vi "Inverse Dynamics (Point).vi"(0 "serial arm in":refnum<class "NI_Robotics_Serial Robot Arm.lvclass">, 1 "external force":dbl[](array[numeric])=[0.0, 0.0, 0.0, 0.0, 0.0, 0.0], 2 "gravity":dbl[](array[numeric]), 5 "joint positions":dbl[](array[numeric]), 7 "joint velocities":dbl[](array[numeric]), 9 "joint accelerations":dbl[](array[numeric]), 11 "error in (no error)":errorcluster) -> (4 "serial arm out":refnum<class "NI_Robotics_Serial Robot Arm.lvclass">, 6 "required torques":dbl[](array[numeric]), 15 "error out":errorcluster)   [LabVIEW 2017, in "NI_Kinematics.lvlib"]
doc: "Returns the amount of torque required for the robotic arm to achieve the joint positions, velocities, and accelerations you specify. Wire data to the <B>joint positions</B> input to determine the polymorphic instance to use or manually select the instance.\n\n<B>.m file:</B> rne"
uses:
  <vilib>/robotics/Kinematics/NI_Kinematics.lvlib
  <vilib>/robotics/Kinematics/Robot/NI_Robotics_Serial Robot Arm.lvclass
  <vilib>/Analysis/Matrix/Datatypes/RealMatrix.ctl
  <vilib>/robotics/Kinematics/Link/Joint Type.ctl
  <vilib>/Analysis/baseanly.llb/Real A x B.vi
  <vilib>/Analysis/baseanly.llb/A x Vector.vi
  <vilib>/Analysis/baseanly.llb/Real Dot Product.vi
  <vilib>/Analysis/Matrix/Numeric/Conversions/Array To Matrix - RA2.vi
  <vilib>/robotics/Kinematics/Link/NI_Robotics_Link.lvclass
  <vilib>/Analysis/NI_AALBase.lvlib
  <vilib>/Analysis/NI_AALPro.lvlib
  <vilib>/Analysis/Matrix/NI_Matrix.lvlib
  <vilib>/robotics/Utilities/NI_Robotics Utilities.lvlib
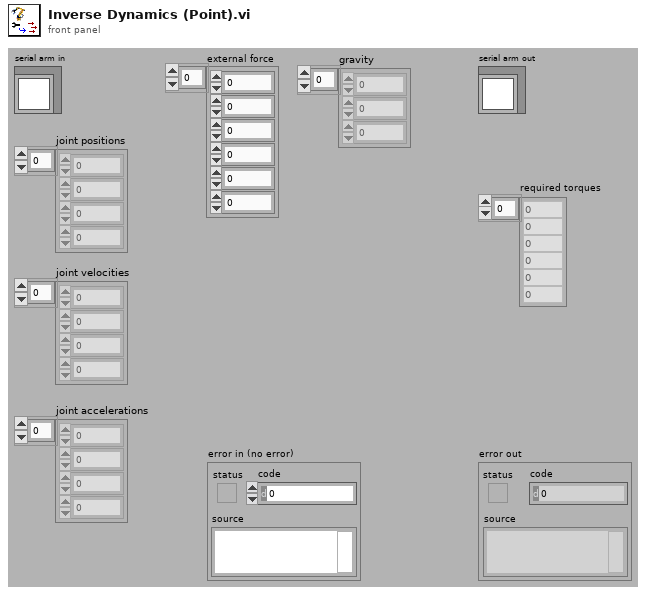
[diagram p1: front panel]
types:
  T1 = typedef "NI_Matrix.lvlib/RealMatrix.ctl" = dbl[][]
  T2 = typedef "NI_Robotics_Link.lvclass/Joint Type.ctl" = enum16{"Revolute", "Prismatic"}
  T3 = typedef "NI_Kinematics.lvlib/DH Convention.ctl" = enum16{"Standard", "Modified"}
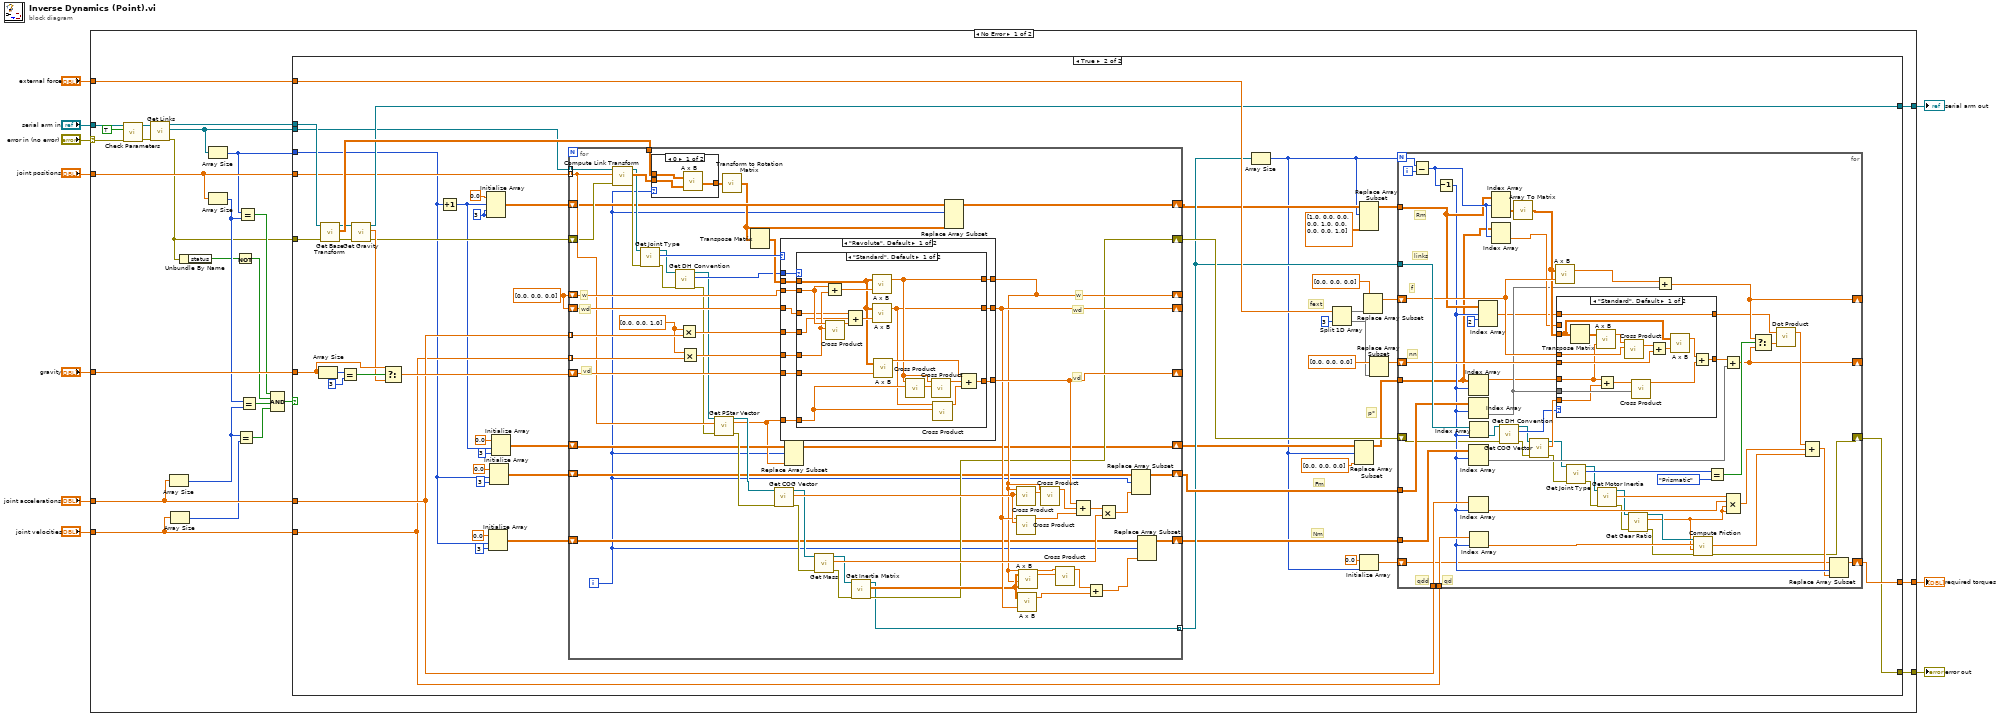
[diagram p0: block diagram]
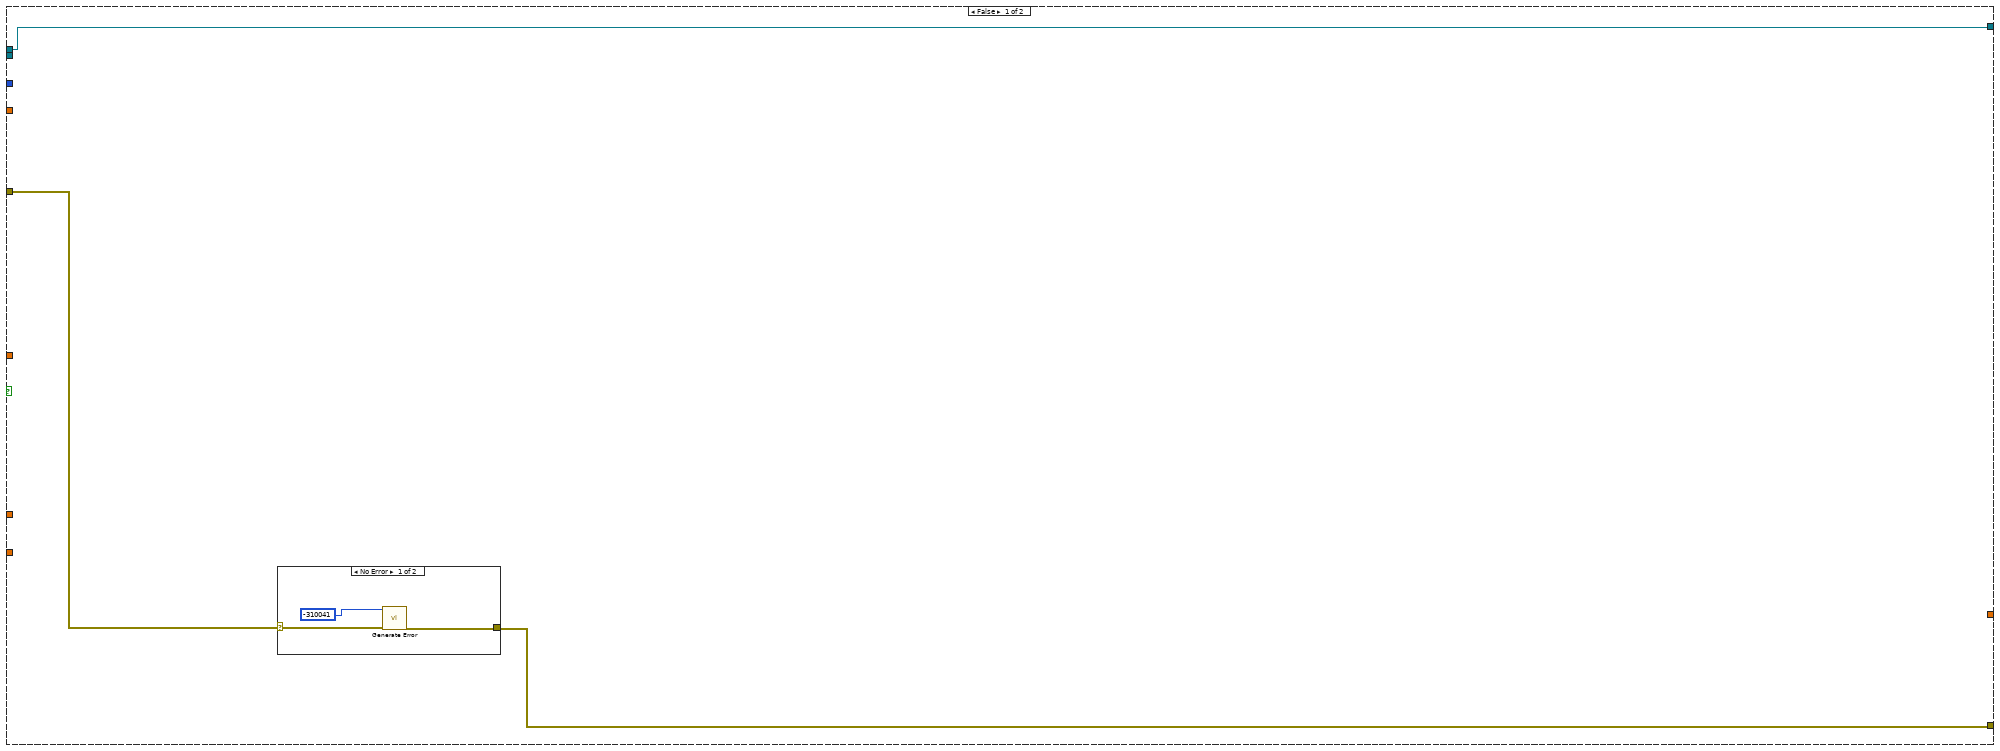
[diagram p2: hidden frame]
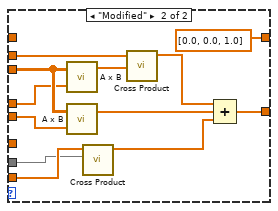
[diagram p4: hidden frame]
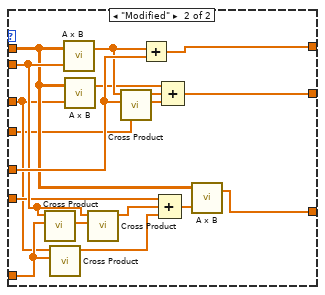
[diagram p5: hidden frame]
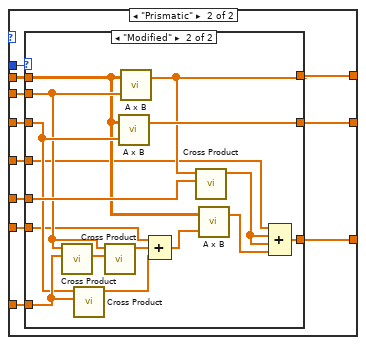
[diagram p6: hidden frame]
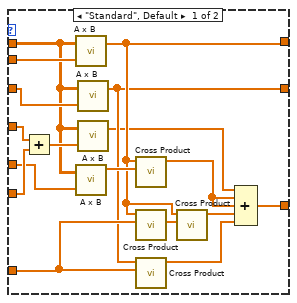
[diagram p7: hidden frame]
diagram:
  n1 = case shown="No Error" "error in (no error)" {
    selector: "error in (no error)" -> [w12 w331]
    tunnel: "external force" -> [w36 _]
    tunnel: [w35 _] -> w9
    tunnel: "gravity" -> [w34 _]
    tunnel: [w32 w332] -> w7
    tunnel: "joint positions" -> [w31 _]
    tunnel: "joint accelerations" -> [w30 _]
    tunnel: "joint velocities" -> [w29 _]
    tunnel: [w23 w331] -> w3
    tunnel: "serial arm in" -> [w17 w332]
    frame No Error {
      n2 = call <vilib>:"Check Parameters.vi"("error in (no error)"=w12, "Dynamic Model"=TRUE, "NI_Robotics_Serial Robot Arm in"=w17) -> ("error out"=w15:errorcluster, "NI_Robotics_Serial Robot Arm out"=w16:refnum<class "NI_Robotics_Serial Robot Arm.lvclass">)  [unwired: 7 in]
      n3 = call <vilib>:"Get Links.vi"("error in (no error)"=w15, "serial arm in"=w16) -> ("error out"=w14:errorcluster, "links"=w28:refnum<class "NI_Robotics_Link.lvclass">[], "serial arm out"=w33:refnum<class "NI_Robotics_Serial Robot Arm.lvclass">)  [unwired: 7 in]
      n4 = Array Size(array=w30) -> (size(s)=w25:i32)
      n5 = Array Size(array=w29) -> (size(s)=w27:i32)
      n6 = Unbundle By Name(w14) -> ("status"=w20:bool)
      n7 = Array Size(array=w31) -> (size(s)=w26:i32)
      n8 = Array Size(array=w28) -> (size(s)=w11:i32)
      n9 = Not(x=w20) -> (.not. x?=w19:bool)
      n10 = Equal?(x=w25, y=w27) -> (x = y?=w22:bool)
      n11 = Equal?(x=w11, y=w26) -> (x = y?=w18:bool)
      n12 = Equal?(x=w26, y=w25) -> (x = y?=w21:bool)
      n13 = Compound Arithmetic op=AND(w18, w19, w21, w22) -> (w24:bool)
      n14 = case shown="True" w24 {
        tunnel: w36 -> [_ w97]
        tunnel: [_ w93] -> w35
        tunnel: w34 -> [_ w89]
        tunnel: w33 -> [w39 w85]
        tunnel: [w39 w83] -> w32
        tunnel: w31 -> [_ w82]
        tunnel: w30 -> [_ w81]
        tunnel: w29 -> [_ w80]
        tunnel: w28 -> [_ w79]
        tunnel: [w37 w74] -> w23
        tunnel: w14 -> [w38 w78]
        tunnel: w11 -> [_ w64]
        frame False {
          n15 = case shown="No Error" w38 {
            selector: w38 -> [w42 w43]
            tunnel: [w41 w43] -> w37
            frame No Error {
              n16 = call <vilib>:"Generate Error.vi"("error in (no error)"=w42, "code"=-310041) -> ("error out"=w41:errorcluster)  [unwired: 9 in]
            }
            frame Error {
              # "propagate error"
            }
          }
        }
        frame True {
          w72 = 3 ("dimension size")
          w98 = dbl[] [0.0, 0.0, 0.0]
          # "fext"
          # "p*"
          # "Nm"
          # "Fm"
          n17 = Array Size(array=w89) -> (size(s)=w91:i32)
          n18 = call <vilib>:"Get Base Transform.vi"("error in (no error)"=w78, "serial arm in"=w85) -> ("error out"=w77:errorcluster, "base transform"=w87:T1, "serial arm out"=w84:refnum<class "NI_Robotics_Serial Robot Arm.lvclass">)  [unwired: 7 in]
          n19 = Equal?(x=w91, y=3) -> (x = y?=w92:bool)
          n20 = call <vilib>:"Get Gravity.vi"("error in (no error)"=w77, "serial arm in"=w84) -> ("error out"=w76:errorcluster, "gravity"=w86:dbl[], "serial arm out"=w83:refnum<class "NI_Robotics_Serial Robot Arm.lvclass">)  [unwired: 7 in]
          n21 = Select(t=w89, s=w92, f=w86) -> (s? t:f=w88:dbl[])
          n22 = Increment(x=w64) -> (x+1=w71:i32)
          n23 = Initialize Array(0.0 ("element"), w71, w72, w72) -> (w63:dbl[][][])
          n24 = Initialize Array(0.0 ("element"), w64, 3 ("dimension size")) -> (w59:dbl[][])
          n25 = Initialize Array(0.0 ("element"), w64, 3 ("dimension size")) -> (w61:dbl[][])
          n26 = Initialize Array(0.0 ("element"), w71, 3 ("dimension size")) -> (w62:dbl[][])
          n27 = for {
            tunnel: w82 -> [w211] mode=indexing
            tunnel: w79 -> [w208] mode=indexing
            tunnel: w87 -> [w236]
            shift-right: [w215] -> _
            shift-left: w98 -> [w225]
            shift-right: [w217] -> _
            shift-left: w98 -> [w224]
            shift-right: [w222] -> _
            shift-left: w88 -> [w232]
            tunnel: w80 -> [w230] mode=indexing
            tunnel: w81 -> [w228] mode=indexing
            shift-right: [w195] -> w75
            shift-left: w76 -> [w209]
            shift-right: [w193] -> w50
            shift-left: w63 -> [w194]
            shift-right: [w189] -> w47
            shift-left: w62 -> [w191]
            shift-right: [w186] -> w60
            shift-left: w61 -> [w187]
            shift-right: [w184] -> w57
            shift-left: w59 -> [w185]
            tunnel: [w182] -> w58 mode=indexing
            i -> [w181]
            w227 = dbl[] [0.0, 0.0, 1.0]
            # "vd"
            # "wd"
            # "w"
            # "vd"
            # "wd"
            # "w"
            n28 = call <vilib>:"Compute Link Transform.vi"("error in (no error)"=w209, "q"=w211, "Link in"=w208) -> ("error out"=w205:errorcluster, "Link Transform"=w237:T1, "Link out"=w207:refnum<class "NI_Robotics_Link.lvclass">)  [unwired: 6 out]
            n29 = call <vilib>:"Get Joint Type.vi"("error in (no error)"=w205, "Link in"=w207) -> ("error out"=w203:errorcluster, "Joint Type"=w234:T2, "Link out"=w206:refnum<class "NI_Robotics_Link.lvclass">)  [unwired: 7 in]
            n30 = case shown="0" w181 {
              tunnel: w237 -> [w328 w330]
              tunnel: [w327 w330] -> w235
              tunnel: w236 -> [w329 _]
              frame 0 {
                n31 = call-poly <vilib>:"A x B.vi"("B"=w328, "A"=w329) -> ("A x B"=w327:T1)  [unwired: 1 out]
              }
              frame 1, Default {
              }
            }
            n32 = call <vilib>:"Get DH Convention.vi"("error in (no error)"=w203, "Link In"=w206) -> ("error out"=w202:errorcluster, "DH Convention"=w210:T3, "Link Out"=w204:refnum<class "NI_Robotics_Link.lvclass">)  [unwired: 7 in]
            n33 = Multiply(x=w227, y=w228) -> (x*y=w229:dbl[])
            n34 = Multiply(x=w227, y=w230) -> (x*y=w231:dbl[])
            n35 = call <vilib>:"Get PStar Vector.vi"("error in (no error)"=w202, "q"=w211, "link in"=w204) -> ("error out"=w198:errorcluster, "p*"=w190:dbl[], "link out"=w201:refnum<class "NI_Robotics_Link.lvclass">)  [unwired: 6 in]
            n36 = call <vilib>:"Transform to Rotation Matrix.vi"("transform"=w235) -> ("rotation matrix"=w192:T1)
            n37 = Transpose Matrix(1:w192) -> (0:w233:T1)
            n38 = call <vilib>:"Get COG Vector.vi"("error in (no error)"=w198, "Link.lvclass in"=w201) -> ("error out"=w197:errorcluster, "COG Vector"=w223:dbl[], "Link.lvclass out"=w200:refnum<class "NI_Robotics_Link.lvclass">)  [unwired: 7 in]
            n39 = case shown="\"Revolute\", Default" w234 {
              tunnel: w233 -> [w246 w288]
              tunnel: w225 -> [w248 w289]
              tunnel: w224 -> [w243 w290]
              tunnel: [w240 w285] -> w215
              tunnel: [w239 w284] -> w217
              tunnel: w229 -> [w242 w291]
              tunnel: w231 -> [w244 w287]
              tunnel: w232 -> [w245 w292]
              tunnel: w190 -> [w241 w286]
              tunnel: [w247 w293] -> w222
              tunnel: w210 -> [w238 w283]
              frame "Revolute", Default {
                n40 = case shown="\"Standard\", Default" w238 {
                  tunnel: w248 -> [w262 w275]
                  tunnel: [w261 w274] -> w247
                  tunnel: w246 -> [w258 w273]
                  tunnel: w245 -> [w257 w271]
                  tunnel: w244 -> [w256 w279]
                  tunnel: w243 -> [w255 w269]
                  tunnel: w242 -> [w254 w266]
                  tunnel: w241 -> [w252 w281]
                  tunnel: [w250 w280] -> w240
                  tunnel: [w249 w278] -> w239
                  frame "Standard", Default {
                    n41 = Add(x=w262, y=w256) -> (x+y=w263:dbl[])
                    n42 = call <vilib>:"Cross Product.vi"("B Vector"=w256, "A Vector"=w262) -> ("Cross Product"=w264:dbl[])  [unwired: 8 in, 1 out]
                    n43 = Compound Arithmetic op=ADD(w255, w254, w264) -> (w265:dbl[])
                    n44 = call-poly <vilib>:"A x B.vi"("Vector"=w263, "A"=w258) -> ("A x Vector"=w250:dbl[])  [unwired: 1 out]
                    n45 = call-poly <vilib>:"A x B.vi"("Vector"=w265, "A"=w258) -> ("A x Vector"=w249:dbl[])  [unwired: 1 out]
                    n46 = call-poly <vilib>:"A x B.vi"("Vector"=w257, "A"=w258) -> ("A x Vector"=w259:dbl[])  [unwired: 1 out]
                    n47 = call <vilib>:"Cross Product.vi"("B Vector"=w252, "A Vector"=w250) -> ("Cross Product"=w253:dbl[])  [unwired: 8 in, 1 out]
                    n48 = call <vilib>:"Cross Product.vi"("B Vector"=w253, "A Vector"=w250) -> ("Cross Product"=w251:dbl[])  [unwired: 8 in, 1 out]
                    n49 = call <vilib>:"Cross Product.vi"("B Vector"=w252, "A Vector"=w249) -> ("Cross Product"=w260:dbl[])  [unwired: 8 in, 1 out]
                    n50 = Compound Arithmetic op=ADD(w259, w251, w260) -> (w261:dbl[])
                  }
                  frame "Modified" {
                    n51 = call <vilib>:"Cross Product.vi"("B Vector"=w281, "A Vector"=w275) -> ("Cross Product"=w282:dbl[])  [unwired: 8 in, 1 out]
                    n52 = call <vilib>:"Cross Product.vi"("B Vector"=w281, "A Vector"=w269) -> ("Cross Product"=w268:dbl[])  [unwired: 8 in, 1 out]
                    n53 = call-poly <vilib>:"A x B.vi"("Vector"=w275, "A"=w273) -> ("A x Vector"=w277:dbl[])  [unwired: 1 out]
                    n54 = call-poly <vilib>:"A x B.vi"("Vector"=w269, "A"=w273) -> ("A x Vector"=w276:dbl[])  [unwired: 1 out]
                    n55 = call <vilib>:"Cross Product.vi"("B Vector"=w282, "A Vector"=w275) -> ("Cross Product"=w270:dbl[])  [unwired: 8 in, 1 out]
                    n56 = call <vilib>:"Cross Product.vi"("B Vector"=w279, "A Vector"=w277) -> ("Cross Product"=w267:dbl[])  [unwired: 8 in, 1 out]
                    n57 = Add(x=w277, y=w279) -> (x+y=w280:dbl[])
                    n58 = Compound Arithmetic op=ADD(w271, w270, w268) -> (w272:dbl[])
                    n59 = Compound Arithmetic op=ADD(w276, w267, w266) -> (w278:dbl[])
                    n60 = call-poly <vilib>:"A x B.vi"("Vector"=w272, "A"=w273) -> ("A x Vector"=w274:dbl[])  [unwired: 1 out]
                  }
                }
              }
              frame "Prismatic" {
                n61 = case shown="\"Modified\"" w283 {
                  tunnel: [w310 w326] -> w293
                  tunnel: w292 -> [w309 w313]
                  tunnel: w291 -> [w308 w314]
                  tunnel: w290 -> [w306 w321]
                  tunnel: w289 -> [w305 w320]
                  tunnel: w288 -> [w303 w319]
                  tunnel: w287 -> [w302 w322]
                  tunnel: w286 -> [w300 w324]
                  tunnel: [w299 w317] -> w285
                  tunnel: [w298 w323] -> w284
                  frame "Standard", Default {
                    n62 = Add(x=w308, y=w309) -> (x+y=w307:dbl[])
                    n63 = call-poly <vilib>:"A x B.vi"("Vector"=w305, "A"=w303) -> ("A x Vector"=w299:dbl[])  [unwired: 1 out]
                    n64 = call-poly <vilib>:"A x B.vi"("Vector"=w302, "A"=w303) -> ("A x Vector"=w304:dbl[])  [unwired: 1 out]
                    n65 = call-poly <vilib>:"A x B.vi"("Vector"=w306, "A"=w303) -> ("A x Vector"=w298:dbl[])  [unwired: 1 out]
                    n66 = call-poly <vilib>:"A x B.vi"("Vector"=w307, "A"=w303) -> ("A x Vector"=w294:dbl[])  [unwired: 1 out]
                    n67 = call <vilib>:"Cross Product.vi"("B Vector"=w304, "A Vector"=w299) -> ("Cross Product"=w295:dbl[])  [unwired: 8 in, 1 out]
                    n68 = call <vilib>:"Cross Product.vi"("B Vector"=w300, "A Vector"=w299) -> ("Cross Product"=w301:dbl[])  [unwired: 8 in, 1 out]
                    n69 = call <vilib>:"Cross Product.vi"("B Vector"=w300, "A Vector"=w298) -> ("Cross Product"=w297:dbl[])  [unwired: 8 in, 1 out]
                    n70 = call <vilib>:"Cross Product.vi"("B Vector"=w301, "A Vector"=w299) -> ("Cross Product"=w296:dbl[])  [unwired: 8 in, 1 out]
                    n71 = Compound Arithmetic op=ADD(w294, w295, w295, w296, w297) -> (w310:dbl[])
                  }
                  frame "Modified" {
                    n72 = call <vilib>:"Cross Product.vi"("B Vector"=w324, "A Vector"=w320) -> ("Cross Product"=w325:dbl[])  [unwired: 8 in, 1 out]
                    n73 = call <vilib>:"Cross Product.vi"("B Vector"=w324, "A Vector"=w321) -> ("Cross Product"=w315:dbl[])  [unwired: 8 in, 1 out]
                    n74 = call <vilib>:"Cross Product.vi"("B Vector"=w325, "A Vector"=w320) -> ("Cross Product"=w316:dbl[])  [unwired: 8 in, 1 out]
                    n75 = call-poly <vilib>:"A x B.vi"("Vector"=w321, "A"=w319) -> ("A x Vector"=w323:dbl[])  [unwired: 1 out]
                    n76 = call-poly <vilib>:"A x B.vi"("Vector"=w320, "A"=w319) -> ("A x Vector"=w317:dbl[])  [unwired: 1 out]
                    n77 = Compound Arithmetic op=ADD(w313, w316, w315) -> (w318:dbl[])
                    n78 = call <vilib>:"Cross Product.vi"("B Vector"=w322, "A Vector"=w317) -> ("Cross Product"=w311:dbl[])  [unwired: 8 in, 1 out]
                    n79 = call-poly <vilib>:"A x B.vi"("Vector"=w318, "A"=w319) -> ("A x Vector"=w312:dbl[])  [unwired: 1 out]
                    n80 = Compound Arithmetic op=ADD(w314, w311, w311, w312) -> (w326:dbl[])
                  }
                }
              }
            }
            n81 = Replace Array Subset(array=w191, new element=w190, index (row)=w181) -> (w189:dbl[][])  [unwired: 1 in]
            n82 = call <vilib>:"Get Mass.vi"("error in (no error)"=w197, "Link in"=w200) -> ("error out"=w196:errorcluster, "Mass"=w219:dbl, "Link out"=w199:refnum<class "NI_Robotics_Link.lvclass">)  [unwired: 7 in]
            n83 = call <vilib>:"Get Inertia Matrix.vi"("error in (no error)"=w196, "Link"=w199) -> ("error out"=w195:errorcluster, "Inertia Matrix"=w216:T1, "Link 2"=w182:refnum<class "NI_Robotics_Link.lvclass">)  [unwired: 7 in]
            n84 = Replace Array Subset(array=w194, new element=w192, index (dim 0)=w181) -> (w193:dbl[][][])  [unwired: 2 in]
            n85 = call <vilib>:"Cross Product.vi"("B Vector"=w223, "A Vector"=w215) -> ("Cross Product"=w226:dbl[])  [unwired: 8 in, 1 out]
            n86 = call <vilib>:"Cross Product.vi"("B Vector"=w223, "A Vector"=w217) -> ("Cross Product"=w220:dbl[])  [unwired: 8 in, 1 out]
            n87 = call-poly <vilib>:"A x B.vi"("Vector"=w217, "A"=w216) -> ("A x Vector"=w213:dbl[])  [unwired: 1 out]
            n88 = call-poly <vilib>:"A x B.vi"("Vector"=w215, "A"=w216) -> ("A x Vector"=w214:dbl[])  [unwired: 1 out]
            n89 = call <vilib>:"Cross Product.vi"("B Vector"=w226, "A Vector"=w215) -> ("Cross Product"=w221:dbl[])  [unwired: 8 in, 1 out]
            n90 = call <vilib>:"Cross Product.vi"("B Vector"=w214, "A Vector"=w215) -> ("Cross Product"=w212:dbl[])  [unwired: 8 in, 1 out]
            n91 = Compound Arithmetic op=ADD(w222, w221, w220) -> (w218:dbl[])
            n92 = Add(x=w212, y=w213) -> (x+y=w183:dbl[])
            n93 = Multiply(x=w218, y=w219) -> (x*y=w188:dbl[])
            n94 = Replace Array Subset(array=w187, new element=w188, index (row)=w181) -> (w186:dbl[][])  [unwired: 1 in]
            n95 = Replace Array Subset(array=w185, new element=w183, index (row)=w181) -> (w184:dbl[][])  [unwired: 1 in]
          }
          n96 = Array Size(array=w58) -> (size(s)=w44:i32)
          n97 = Split 1D Array(array=w97, index=3) -> (first subarray=w55:dbl[], second subarray=w51:dbl[])
          n98 = Replace Array Subset(array=w47, new element=dbl[] [0.0, 0.0, 0.0], index (row)=w44) -> (w46:dbl[][])  [unwired: 1 in]
          n99 = Replace Array Subset(array=w50, new element=T1 [[1.0, 0.0, 0.0], [0.0, 1.0, 0.0], [0.0, 0.0, 1.0]] ("Real Matrix"), index (dim 0)=w44) -> (w49:dbl[][][])  [unwired: 2 in]
          n100 = Initialize Array(0.0 ("element"), w44) -> (w94:dbl[])
          n101 = Replace Array Subset(array=dbl[] [0.0, 0.0, 0.0], new element=w55) -> (w54:dbl[])  [unwired: 1 in]
          n102 = Replace Array Subset(array=dbl[] [0.0, 0.0, 0.0], new element=w51) -> (w53:dbl[])  [unwired: 1 in]
          n103 = for {
            N: w44 -> [w153]
            tunnel: w49 -> [w143]
            tunnel: w58 -> [w151]
            tunnel: w46 -> [w115]
            shift-right: [w130] -> _
            shift-left: w53 -> [w145]
            shift-right: [w141] -> _
            shift-left: w54 -> [w146]
            tunnel: w60 -> [w149]
            tunnel: w57 -> [w148]
            shift-right: [w142] -> w93
            shift-left: w94 -> [w114]
            tunnel: w81 -> [w139]
            tunnel: w80 -> [w138]
            shift-right: [w102] -> w74
            shift-left: w75 -> [w111]
            i -> [w152]
            # "qd"
            # "qdd"
            # "f"
            # "nn"
            # "Rm"
            # "links"
            n104 = Subtract(x=w153, y=w152) -> (x-y=w150:i32)
            n105 = Decrement(x=w150) -> (x-1=w137:i32)
            n106 = Index Array(array=w115, index (row)=w137) -> (element=w116:dbl[])  [unwired: 1 in]
            n107 = Index Array(array=w149, index (row)=w137) -> (element=w124:dbl[])  [unwired: 1 in]
            n108 = Index Array(array=w148, index (row)=w137) -> (element=w131:dbl[])  [unwired: 1 in]
            n109 = Index Array(array=w139, index=w137) -> (element=w118:dbl)
            n110 = Index Array(array=w151, index=w137) -> (element=w126:refnum<class "NI_Robotics_Link.lvclass">)
            n111 = Index Array(array=w138, index=w137) -> (element=w136:dbl)
            n112 = Index Array(array=w143, index (dim 0)=w137, index (dim 1)=2 ("index (row)")) -> (element=w120:dbl[])  [unwired: 1 in]
            n113 = Index Array(array=w143, index (dim 0)=w150) -> (element=w101:dbl[][])  [unwired: 2 in]
            n114 = Index Array(array=w115, index (row)=w150) -> (element=w125:dbl[])  [unwired: 1 in]
            n115 = call <vilib>:"Get DH Convention.vi"("error in (no error)"=w111, "Link In"=w126) -> ("error out"=w112:errorcluster, "DH Convention"=w127:T3, "Link Out"=w113:refnum<class "NI_Robotics_Link.lvclass">)  [unwired: 7 in]
            n116 = call-poly <vilib>:"Array To Matrix.vi"("Real 2D Array"=w101) -> ("Real Matrix"=w144:T1)
            n117 = call <vilib>:"Get COG Vector.vi"("error in (no error)"=w112, "Link.lvclass in"=w113) -> ("error out"=w109:errorcluster, "COG Vector"=w128:dbl[], "Link.lvclass out"=w110:refnum<class "NI_Robotics_Link.lvclass">)  [unwired: 7 in]
            n118 = call-poly <vilib>:"A x B.vi"("Vector"=w146, "A"=w144) -> ("A x Vector"=w147:dbl[])  [unwired: 1 out]
            n119 = case shown="\"Standard\", Default" w127 {
              tunnel: w146 -> [w167 w175]
              tunnel: w145 -> [w166 w180]
              tunnel: w144 -> [w155 w176]
              tunnel: w116 -> [w156 _]
              tunnel: w124 -> [w163 w177]
              tunnel: [w158 w179] -> w129
              tunnel: w128 -> [w157 w178]
              tunnel: w125 -> [_ w170]
              tunnel: w120 -> [w154 _]
              tunnel: [w154 dbl[] [0.0, 0.0, 1.0]] -> w119
              frame "Standard", Default {
                n120 = Transpose Matrix(1:w155) -> (0:w161:T1)
                n121 = call-poly <vilib>:"A x B.vi"("Vector"=w156, "A"=w161) -> ("A x Vector"=w168:dbl[])  [unwired: 1 out]
                n122 = Add(x=w156, y=w157) -> (x+y=w162:dbl[])
                n123 = call <vilib>:"Cross Product.vi"("B Vector"=w167, "A Vector"=w168) -> ("Cross Product"=w165:dbl[])  [unwired: 8 in, 1 out]
                n124 = call <vilib>:"Cross Product.vi"("B Vector"=w163, "A Vector"=w162) -> ("Cross Product"=w159:dbl[])  [unwired: 8 in, 1 out]
                n125 = Add(x=w165, y=w166) -> (x+y=w164:dbl[])
                n126 = call-poly <vilib>:"A x B.vi"("Vector"=w164, "A"=w155) -> ("A x Vector"=w160:dbl[])  [unwired: 1 out]
                n127 = Add(x=w160, y=w159) -> (x+y=w158:dbl[])
              }
              frame "Modified" {
                n128 = call-poly <vilib>:"A x B.vi"("Vector"=w175, "A"=w176) -> ("A x Vector"=w172:dbl[])  [unwired: 1 out]
                n129 = call-poly <vilib>:"A x B.vi"("Vector"=w180, "A"=w176) -> ("A x Vector"=w173:dbl[])  [unwired: 1 out]
                n130 = call <vilib>:"Cross Product.vi"("B Vector"=w177, "A Vector"=w178) -> ("Cross Product"=w174:dbl[])  [unwired: 8 in, 1 out]
                n131 = call <vilib>:"Cross Product.vi"("B Vector"=w172, "A Vector"=w170) -> ("Cross Product"=w171:dbl[])  [unwired: 8 in, 1 out]
                n132 = Compound Arithmetic op=ADD(w171, w173, w174) -> (w179:dbl[])
              }
            }
            n133 = call <vilib>:"Get Joint Type.vi"("error in (no error)"=w109, "Link in"=w110) -> ("error out"=w107:errorcluster, "Joint Type"=w122:T2, "Link out"=w108:refnum<class "NI_Robotics_Link.lvclass">)  [unwired: 7 in]
            n134 = call <vilib>:"Get Motor Inertia.vi"("error in (no error)"=w107, "Link in"=w108) -> ("error out"=w105:errorcluster, "Motor Inertia"=w117:dbl, "Link out"=w106:refnum<class "NI_Robotics_Link.lvclass">)  [unwired: 7 in]
            n135 = call <vilib>:"Get Gear Ratio.vi"("error in (no error)"=w105, "Link In"=w106) -> ("error out"=w103:errorcluster, "Gear Ratio"=w99:dbl, "Link Out"=w104:refnum<class "NI_Robotics_Link.lvclass">)  [unwired: 7 in]
            n136 = Add(x=w147, y=w124) -> (x+y=w141:dbl[])
            n137 = call <vilib>:"Compute Friction.vi"("error in (no error)"=w103, "gear ratio"=w99, "qd"=w136, "link in"=w104) -> ("error out"=w102:errorcluster, "Friction"=w100:dbl)  [unwired: 5 in, 1 out]
            n138 = Equal?(x=w122, y=Joint_Type."Prismatic") -> (x = y?=w140:bool)
            n139 = Add(x=w129, y=w131) -> (x+y=w130:dbl[])
            n140 = Compound Arithmetic op=MULTIPLY(w117, w118, w99, w99) -> (w133:dbl)
            n141 = Select(t=w141, s=w140, f=w130) -> (s? t:f=w132:dbl[])
            n142 = call-poly <vilib>:"Dot Product.vi"("Y Vector"=w132, "X Vector"=w119) -> ("X * Y"=w134:dbl)  [unwired: 1 out]
            n143 = Compound Arithmetic op=ADD(w134, w133, w100) -> (w135:dbl)
            n144 = Replace Array Subset(array=w114, new element=w135, index=w137) -> (w142:dbl[])
          }
        }
      }
    }
    frame Error {
    }
  }
  "serial arm out" <- w7
  "required torques" <- w9
  "error out" <- w3
